vi "Configure Trigger Power Meter.vi"(0 "VISA resource name":refnum<visa-resource-name>, 1 "Trigger Level (0 dBm)":dbl, 2 "Trigger Hold Off Time (0.01 seconds)":dbl=0.01, 5 "Trigger Type (0: Free Run)":i32(ring) items=["Free Run", "Continuous", "Single"], 7 "Source Type (0: External)":i32(ring) items=["External", "Internal"], 9 "Auto Trigger Level (F: Disable)":bool, 11 "error in (no error)":errorcluster, 12 "Trigger Slope Mode (0: Positive)":i32(ring) items=["Positive", "Negative"], 13 "Trigger Hysteresis Value (1)":dbl=1.0) -> (4 "VISA resource name out":refnum<visa-resource-name>, 15 "error out":errorcluster)   [LabVIEW 2022 SP3, in "Agilent N934X Series.lvlib"]
doc: "Configure the trigger settings of Power Meter Measurement Type.\n\nNote:\nThis VI is only applicable for N9321C, N9322C, N9323C, N9324C models."
uses:
  <instrlib>/Agilent N934X Series/Agilent N934X Series.lvlib
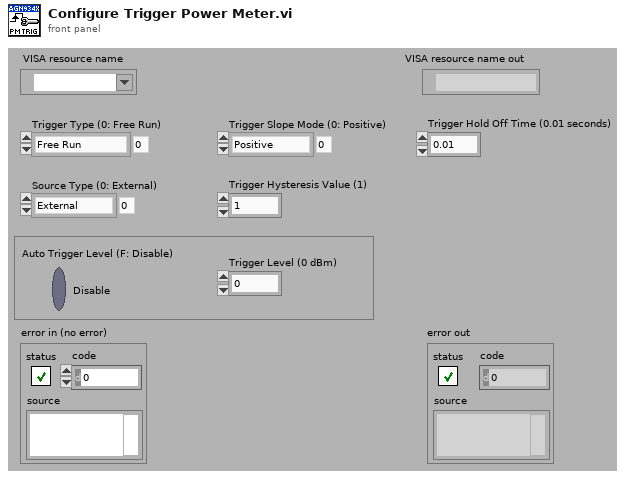
[diagram p1: front panel]
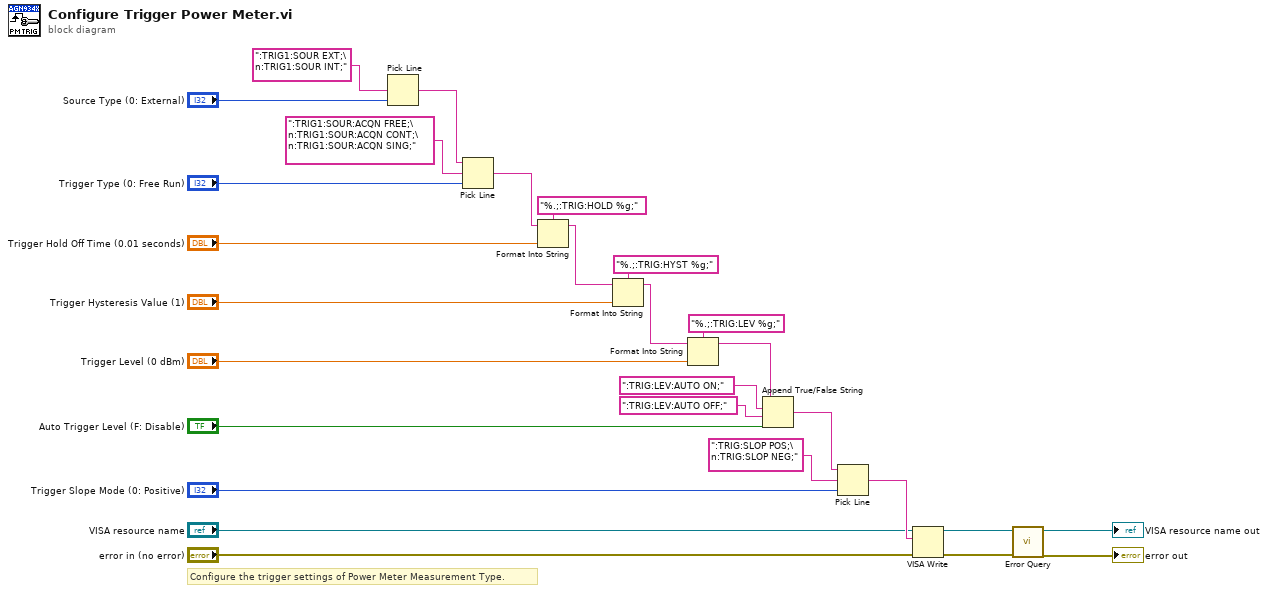
[diagram p0: block diagram]
diagram:
  # "Configure the trigger settings of Power Meter Measurement Type."
  n1 = Pick Line(multi-line string=":TRIG1:SOUR EXT;\n:TRIG1:SOUR INT;", line index="Source Type (0: External)") -> (output string=w24:string)  [unwired: 1 in]
  n2 = Pick Line(string ("")=w24, multi-line string=":TRIG1:SOUR:ACQN FREE;\n:TRIG1:SOUR:ACQN CONT;\n:TRIG1:SOUR:ACQN SING;", line index="Trigger Type (0: Free Run)") -> (output string=w23:string)
  n3 = Format Into String(format string="%.;:TRIG:HOLD %g;", initial string=w23, "Trigger Hold Off Time (0.01 seconds)") -> (resulting string=w20:string)  [unwired: 1 in, 1 out]
  n4 = Format Into String(format string="%.;:TRIG:HYST %g;", initial string=w20, "Trigger Hysteresis Value (1)") -> (resulting string=w17:string)  [unwired: 1 in, 1 out]
  n5 = Format Into String(format string="%.;:TRIG:LEV %g;", initial string=w17, "Trigger Level (0 dBm)") -> (resulting string=w14:string)  [unwired: 1 in, 1 out]
  n6 = Append True/False String(1:"Auto Trigger Level (F: Disable)", 2:":TRIG:LEV:AUTO OFF;", 3:":TRIG:LEV:AUTO ON;", 4:w14) -> (0:w8:string)
  n7 = Pick Line(string ("")=w8, multi-line string=":TRIG:SLOP POS;\n:TRIG:SLOP NEG;", line index="Trigger Slope Mode (0: Positive)") -> (output string=w7:string)
  n8 = VISA Write(VISA resource name="VISA resource name", write buffer=w7, error in (no error)="error in (no error)") -> (VISA resource name out=w4:refnum<visa-resource-name>, error out=w3:errorcluster)  [unwired: 1 out]
  n9 = call <instrlib>:"Error Query.vi"("error in (no error)"=w3, "VISA resource name"=w4) -> ("error out"=→"error out":errorcluster, "VISA resource name out"=→"VISA resource name out":refnum<visa-resource-name>)  [unwired: 6 in, 2 out]
